vi "Crosshairs 2.vi"   [LabVIEW 2012]
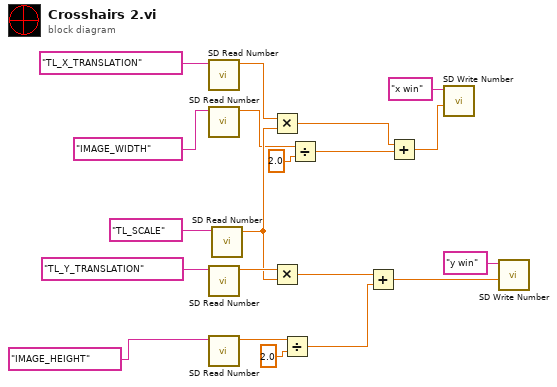
[diagram p0: block diagram]
diagram:
  n1 = call <vilib>:"SD Read Number.vi"("Name"="TL_X_TRANSLATION") -> ("Numeric"=w9:dbl)  [unwired: 8 in, 2 out]
  n2 = call <vilib>:"SD Read Number.vi"("Name"="IMAGE_WIDTH") -> ("Numeric"=w1:dbl)  [unwired: 8 in, 2 out]
  n3 = call <vilib>:"SD Read Number.vi"("Name"="TL_Y_TRANSLATION") -> ("Numeric"=w14:dbl)  [unwired: 8 in, 2 out]
  n4 = call <vilib>:"SD Read Number.vi"("Name"="IMAGE_HEIGHT") -> ("Numeric"=w6:dbl)  [unwired: 8 in, 2 out]
  n5 = call <vilib>:"SD Read Number.vi"("Name"="TL_SCALE") -> ("Numeric"=w12:dbl)  [unwired: 8 in, 2 out]
  n6 = Multiply(x=w9, y=w12) -> (x*y=w4:dbl)
  n7 = Multiply(x=w14, y=w12) -> (x*y=w13:dbl)
  n8 = Divide(x=w6, y=2.0) -> (x/y=w5:dbl)
  n9 = Divide(x=w1, y=2.0) -> (x/y=w3:dbl)
  n10 = Add(x=w13, y=w5) -> (x+y=w18:dbl)
  n11 = Add(x=w4, y=w3) -> (x+y=w2:dbl)
  n12 = call <vilib>:"SD Write Number.vi"("Numeric"=w2, "Name"="x win") -> ()  [unwired: 8 in, 2 out]
  n13 = call <vilib>:"SD Write Number.vi"("Numeric"=w18, "Name"="y win") -> ()  [unwired: 8 in, 2 out]
